vi "Alias Does Not Exist Error.vi"() -> (2 "Error":errorcluster)   [LabVIEW 2021, in "jettl.lvlib" / "jettl Queue Actor.lvlib" / "jettl Queue Actor.lvclass"]
uses:
  jettl Queue Actor.lvclass
  jettl Queue Actor.lvclass/jettl Queue Actor.ctl
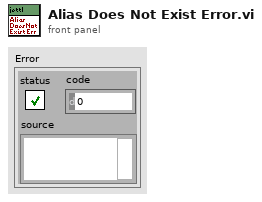
[diagram p1: front panel]
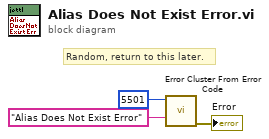
[diagram p0: block diagram]
diagram:
  # "Random, return to this later."
  n1 = call <vilib>:"Error Cluster From Error Code.vi"("error message (\"\")"="Alias Does Not Exist Error" ("error message (\"\")"), "error code (0)"=5501) -> ("error out"=→"Error":errorcluster)  [unwired: 7 in]
